vi "F Dwf Analog In Trigger Channel Info.vi"(8 "error in (no error)":errorcluster, 9 "pidxMax":i32, 10 "pidxMin":i32, 11 "hdwf":i32) -> (0 "error out":errorcluster, 1 "pidxMax out":i32, 2 "pidxMin out":i32, 3 "function return":i32)   [LabVIEW 2019, in "Olasdwf.lvlib"]
doc: "DWFAPI int FDwfAnalogInTriggerChannelInfo(HDWF hdwf, int *pidxMin, int *pidxMax);"
uses:
  Olasdwf.lvlib
  Windows/System32/dwf.dll
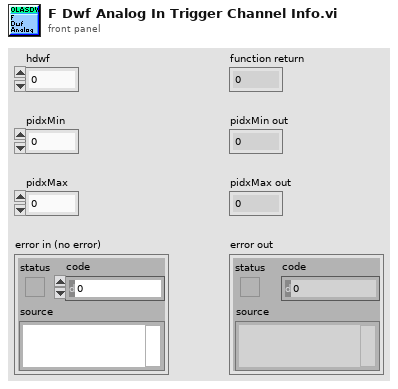
[diagram p1: front panel]
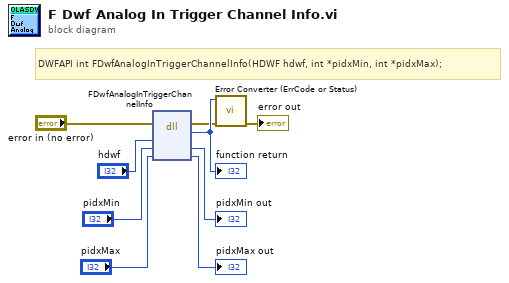
[diagram p0: block diagram]
diagram:
  # "DWFAPI int FDwfAnalogInTriggerChannelInfo(HDWF hdwf, int *pidxMin, int *pidxMax);"
  n1 = dll-call lib="C:/Windows/System32/dwf.*" fn="FDwfAnalogInTriggerChannelInfo"(error in="error in (no error)", "hdwf"="hdwf", "pidxMin"="pidxMin", "pidxMax"="pidxMax") -> (error out=w2:errorcluster, w9:i32, "pidxMin"=→"pidxMin out":i32, "pidxMax"=→"pidxMax out":i32)  [unwired: 3 in, 1 out]
  "function return" <- w9
  n2 = call "Error Converter (ErrCode or Status).vi"("error in (no error)"=w2, "error code"=w9) -> ("error out"=→"error out":errorcluster)  [unwired: 9 in]
